vi "去除背景fin_forfunctionuse.vi"(1 "阈值":i32(slide)=50 scale=0.0..90.0, 2 "Image Src":T1) -> (0 "Image Out":T1)   [LabVIEW 2018]
uses:
  <vilib>/vision/Image Controls.llb/IMAQ Image.ctl
  <vilib>/vision/NI_Vision_Development_Module.lvlib
panel:
  out "Image 2":T1(plugin-control)
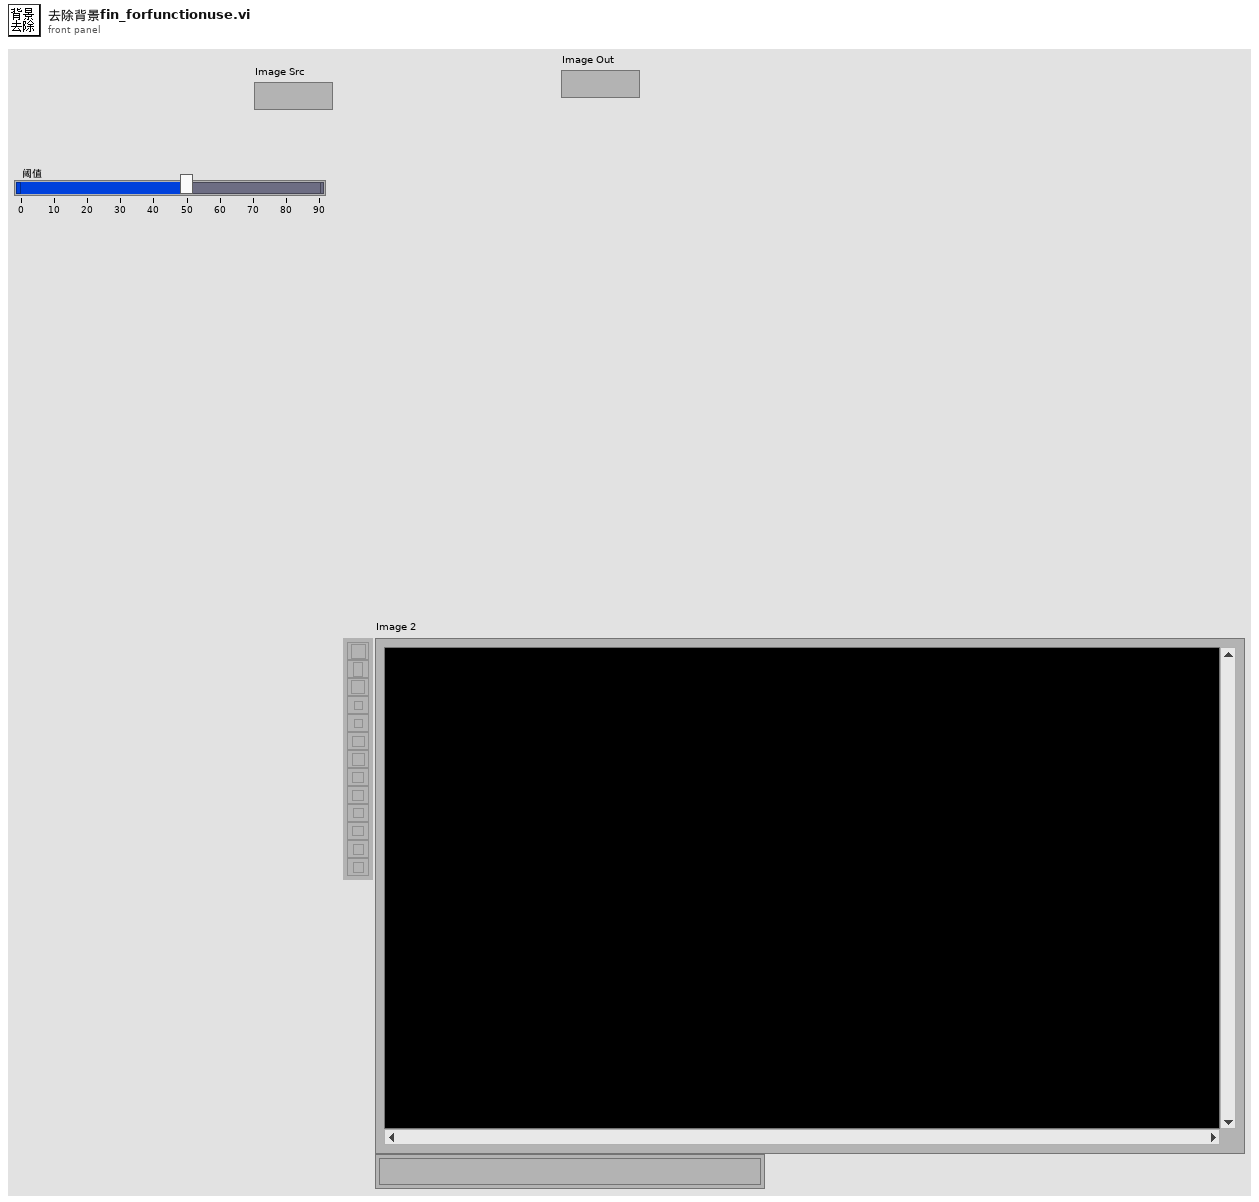
[diagram p1: front panel]
types:
  T1 = typedef "IMAQ Image.ctl" = refnum<image>
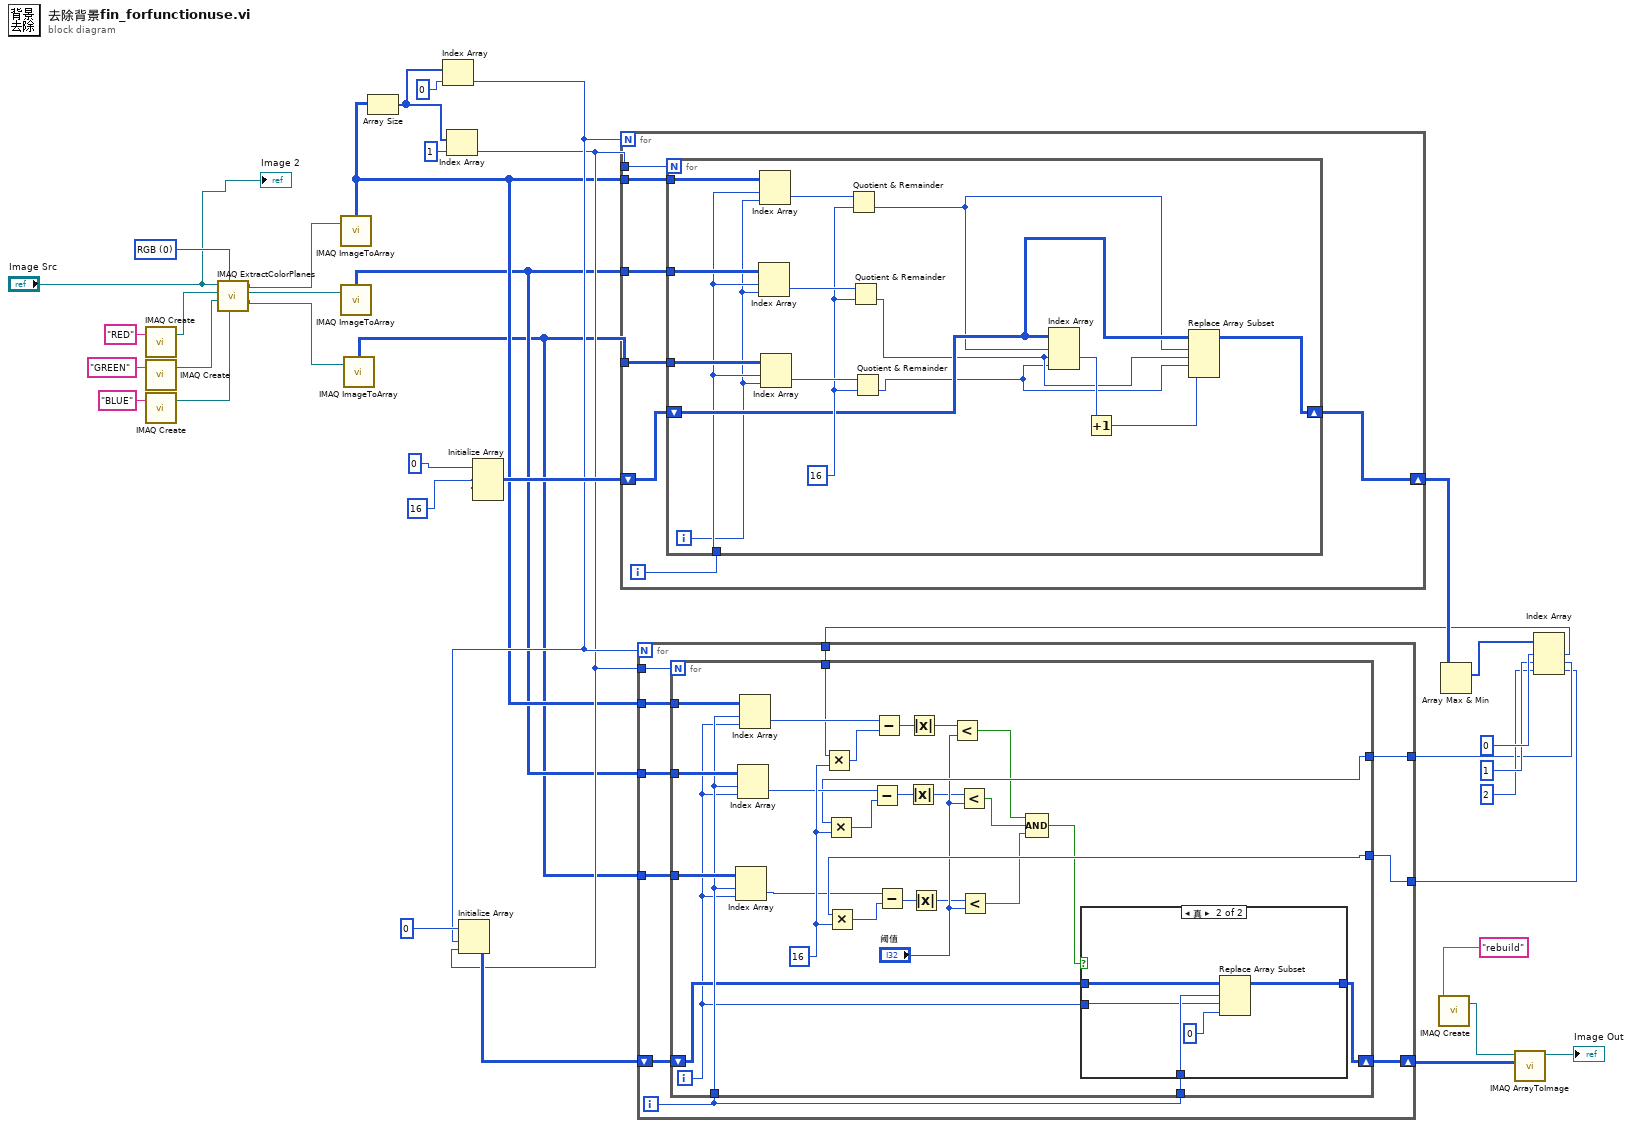
[diagram p0: block diagram]
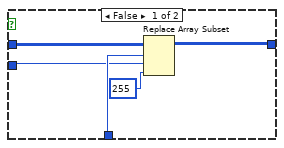
[diagram p2: hidden frame]
diagram:
  w25 = 16
  w36 = u16 0 items=["RGB", "HSL", "HSV", "HSI"] ("Color Mode")
  n1 = call "IMAQ Create"("Image Name"="RED") -> ("New Image"=w30:T1)  [unwired: 4 in, 1 out]
  n2 = call "IMAQ Create"("Image Name"="GREEN") -> ("New Image"=w31:T1)  [unwired: 4 in, 1 out]
  n3 = call "IMAQ Create"("Image Name"="BLUE") -> ("New Image"=w32:T1)  [unwired: 4 in, 1 out]
  n4 = call "IMAQ ExtractColorPlanes"("Blue or Luma or Val or Inten Plane"=w32, "Color Mode"=w36, "Green or Sat Plane"=w31, "Red or Hue Plane"=w30, "Image Src"="Image Src") -> ("Blue or Luma or Val or Inten Plane out"=w27:T1, "Green or Sat Plane out"=w28:T1, "Red or Hue Plane out"=w29:T1)  [unwired: 3 in, 1 out]
  n5 = call "IMAQ ImageToArray"("Image"=w29) -> ("Image Pixels (U8)"=w5:u8[][])  [unwired: 3 in, 4 out]
  n6 = call "IMAQ ImageToArray"("Image"=w28) -> ("Image Pixels (U8)"=w4:u8[][])  [unwired: 3 in, 4 out]
  n7 = call "IMAQ ImageToArray"("Image"=w27) -> ("Image Pixels (U8)"=w3:u8[][])  [unwired: 3 in, 4 out]
  n8 = Array Size(array=w5) -> (size(s)=w21:i32[])
  n9 = Index Array(array=w21, index=0 ("索引")) -> (element=w10:i32)
  n10 = Index Array(array=w21, index=1 ("索引")) -> (element=w9:i32)
  n11 = Initialize Array(0, w10, w9) -> (w11:i32[][])
  n12 = Initialize Array(0, w25, w25, w25) -> (w24:i32[][][])
  n13 = for {
    N: w10 -> [_]
    shift-right: [w42] -> w20
    shift-left: w24 -> [w43]
    tunnel: w9 -> [w40]
    tunnel: w5 -> [w39]
    tunnel: w4 -> [w38]
    tunnel: w3 -> [w37]
    i -> [w41]
    n14 = for {
      N: w40 -> [_]
      shift-right: [w49] -> w42
      shift-left: w43 -> [w51]
      tunnel: w41 -> [w48]
      tunnel: w39 -> [w58]
      tunnel: w38 -> [w57]
      tunnel: w37 -> [w56]
      i -> [w47]
      w53 = 16
      n15 = Index Array(array=w57, index (row)=w48, index (col)=w47) -> (element=w55:u8)
      n16 = Index Array(array=w58, index (row)=w48, index (col)=w47) -> (element=w59:u8)
      n17 = Index Array(array=w56, index (row)=w48, index (col)=w47) -> (element=w54:u8)
      n18 = Quotient & Remainder(x=w59, y=w53) -> (floor(x/y)=w44:i32)  [unwired: 1 out]
      n19 = Quotient & Remainder(x=w55, y=w53) -> (floor(x/y)=w46:i32)  [unwired: 1 out]
      n20 = Quotient & Remainder(x=w54, y=w53) -> (floor(x/y)=w45:i32)  [unwired: 1 out]
      n21 = Index Array(array=w51, index (dim 0)=w44, index (dim 1)=w46, index (dim 2)=w45) -> (element=w52:i32)
      n22 = Increment(x=w52) -> (x+1=w50:i32)
      n23 = Replace Array Subset(array=w51, new element=w50, index (dim 0)=w44, index (dim 1)=w46, index (dim 2)=w45) -> (w49:i32[][][])
    }
  }
  n24 = call "IMAQ Create"("Image Name"="rebuild") -> ("New Image"=w8:T1)  [unwired: 4 in, 1 out]
  n25 = Array Max & Min(array=w20) -> (max index (indices)=w18:i32[])  [unwired: 3 out]
  n26 = Index Array(array=w18, index #1=0 ("索引"), index #2=1 ("索引"), index #3=2 ("索引")) -> (element #1=w14:i32, element #2=w13:i32, element #3=w12:i32)
  n27 = for {
    N: w10 -> [_]
    tunnel: w9 -> [w69]
    tunnel: w5 -> [w68]
    tunnel: w4 -> [w67]
    tunnel: w3 -> [w66]
    tunnel: w14 -> [w65]
    tunnel: w13 -> [w64]
    tunnel: w12 -> [w63]
    shift-right: [w62] -> w6
    shift-left: w11 -> [w61]
    i -> [w60]
    n28 = for {
      N: w69 -> [_]
      tunnel: w68 -> [w98]
      tunnel: w67 -> [w97]
      tunnel: w66 -> [w96]
      tunnel: w60 -> [w95]
      tunnel: w65 -> [w88]
      tunnel: w64 -> [w85]
      tunnel: w63 -> [w83]
      shift-right: [w91] -> w62
      shift-left: w61 -> [w94]
      tunnel: w60 -> [w93]
      i -> [w92]
      w89 = 16
      n29 = Index Array(array=w96, index (row)=w95, index (col)=w92) -> (element=w82:u8)
      n30 = Index Array(array=w97, index (row)=w95, index (col)=w92) -> (element=w86:u8)
      n31 = Index Array(array=w98, index (row)=w95, index (col)=w92) -> (element=w90:u8)
      n32 = Multiply(x=w88, y=w89) -> (x*y=w87:i32)
      n33 = Multiply(x=w85, y=w89) -> (x*y=w84:i32)
      n34 = Multiply(x=w83, y=w89) -> (x*y=w81:i32)
      n35 = Subtract(x=w86, y=w84) -> (x-y=w73:i32)
      n36 = Subtract(x=w90, y=w87) -> (x-y=w75:i32)
      n37 = Subtract(x=w82, y=w81) -> (x-y=w71:i32)
      n38 = Absolute Value(x=w73) -> (abs(x)=w72:i32)
      n39 = Absolute Value(x=w75) -> (abs(x)=w74:i32)
      n40 = Absolute Value(x=w71) -> (abs(x)=w70:i32)
      n41 = Less?(x=w74, y="阈值") -> (x < y?=w79:bool)
      n42 = Less?(x=w72, y="阈值") -> (x < y?=w78:bool)
      n43 = Less?(x=w70, y="阈值") -> (x < y?=w77:bool)
      n44 = Compound Arithmetic op=AND ("复合运算")(w79, w78, w77) -> (w76:bool)
      n45 = case shown="真" w76 {
        tunnel: w94 -> [w103 w108]
        tunnel: w93 -> [w102 w107]
        tunnel: w92 -> [w101 w106]
        tunnel: [w99 w104] -> w91
        frame False {
          n46 = Replace Array Subset(array=w103, new element=255 ("新元素/子数组"), index (row)=w102, index (col)=w101) -> (w99:i32[][])
        }
        frame True {
          n47 = Replace Array Subset(array=w108, new element=0 ("新元素/子数组"), index (row)=w107, index (col)=w106) -> (w104:i32[][])
        }
      }
    }
  }
  n48 = call "IMAQ ArrayToImage"("Image Pixels (U8)"=w6, "Image"=w8) -> ("Image Out"=→"Image Out":T1)  [unwired: 8 in, 1 out]
  "Image 2" <- "Image Src"
